vi "KH_DAQ_TURCK_FGlob_AI Status.vi"(5 "Function (Recall One)":T1=enum."Recall one", 8 "err in":errorcluster caption="error", 9 "AI Unscaled IN":i16[](array[numeric]), 11 "StatusIn":bool[](array[boolean])) -> (0 "err out":errorcluster caption="error", 1 "AI Values out unscaled":i16[](array[numeric]), 3 "StatusOut":bool[](array[boolean]))   [LabVIEW 2021]
uses:
  KH Turck EthernetIP 17.12/KH TURCK TypeDefs FGlob.ctl
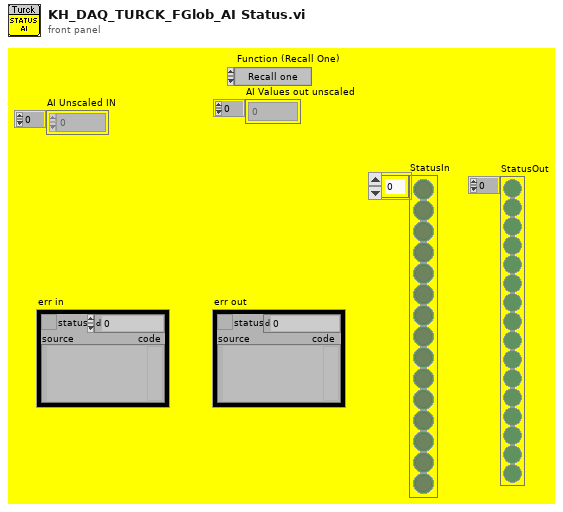
[diagram p1: front panel]
types:
  T1 = typedef "KH TURCK TypeDefs FGlob.ctl" = enum16{"Put one", "Put all", "Recall one", "Recall all"}
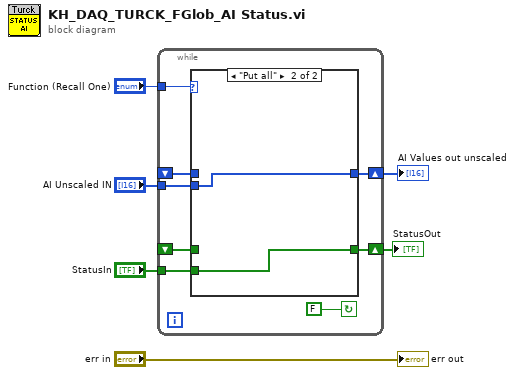
[diagram p0: block diagram]
diagram:
  n1 = while {
    tunnel: "Function (Recall One)" -> [w13]
    shift-right: [w12] -> w4
    shift-left: _ -> [w11]
    tunnel: "AI Unscaled IN" -> [w10]
    tunnel: "StatusIn" -> [w9]
    shift-right: [w8] -> w1
    shift-left: _ -> [w7]
    stop <- FALSE continue-if-true
    n2 = case shown="\"Put all\"" w13 {
      tunnel: [w16 w18] -> w12
      tunnel: w11 -> [w16 _]
      tunnel: w10 -> [_ w18]
      tunnel: w9 -> [_ w17]
      tunnel: [w15 w17] -> w8
      tunnel: w7 -> [w15 _]
      frame "Recall all", Default {
      }
      frame "Put all" {
      }
    }
  }
  "AI Values out unscaled" <- w4
  "StatusOut" <- w1
  "err out" <- "err in"
